vi "MU Read Sens.vi"(8 "error in (no error)":errorcluster, 11 "handle":u64) -> (0 "error out (no error)":errorcluster, 2 "data":T1, 3 "function return":u32)   [LabVIEW 2017, in "MU_3SL_interface.lvlib"]
uses:
  MU_3SL_interface.lvlib
  lib/MU_3SL_interface.dll
panel:
  in  "data":T1
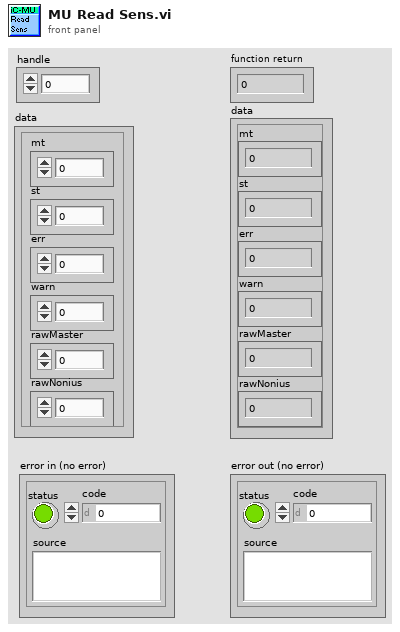
[diagram p1: front panel]
types:
  T1 = cluster{"mt":u32, "st":u32, "err":u32, "warn":u32, "rawMaster":u32, "rawNonius":u32}
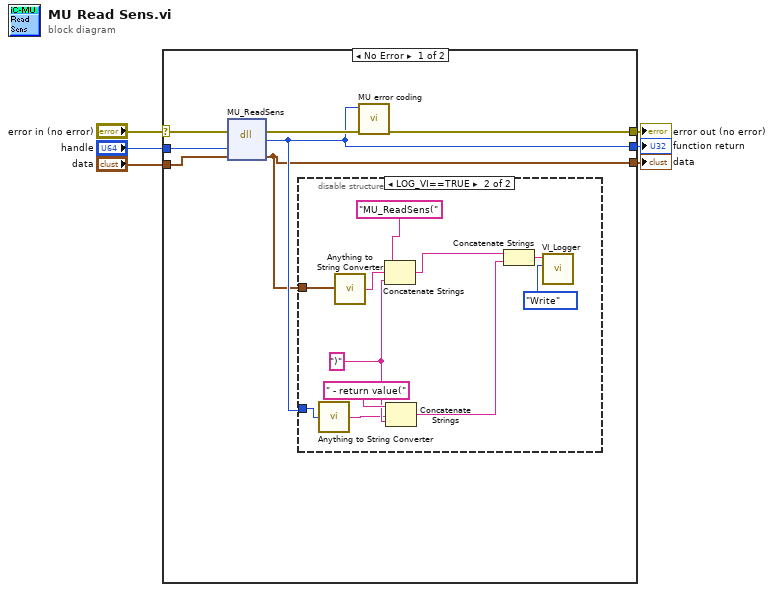
[diagram p0: block diagram]
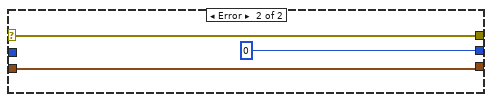
[diagram p3: hidden frame]
diagram:
  n1 = case shown="No Error" "error in (no error)" {
    selector: "error in (no error)" -> [w9 w27]
    tunnel: [w8 u32 0 ("return type")] -> w6
    tunnel: "handle" -> [w13 _]
    tunnel: [w11 w27] -> w4
    tunnel: "data" -> [w10 w25]
    tunnel: [w7 w25] -> w1
    frame No Error {
      n2 = dll-call lib="C:/Users/bes/AppData/Roaming/work/mu_9so/icsubmodules/soft_mu_3sl_master/lv_interface/lib/MU_3SL_interface**.*" fn="MU_ReadSens"(error in=w9, "handle"=w13, "data"=w10) -> (error out=w12:errorcluster, "return type"=w8:u32, "data"=w7:T1)  [unwired: 3 in, 1 out]
      n3 = disable-structure shown="LOG_VI==TRUE" {
        disable-tunnel: w8 -> [_ w16]
        disable-tunnel: w7 -> [_ w18]
        frame condition #0 {
        }
        frame condition #1 (active) {
          w19 = ")" ("string")
          n4 = call "Anything to String Converter.vi"("anything"=w16) -> ("String"=w15:string)
          n5 = call "Anything to String Converter.vi"("anything"=w18) -> ("String"=w17:string)
          n6 = Concatenate Strings("MU_ReadSens(" ("Info in"), w17, w19) -> (w14:string)
          n7 = Concatenate Strings(" - return value(" ("string"), w15, w19) -> (w22:string)
          n8 = Concatenate Strings(w14, w22) -> (w21:string)
          n9 = call "VI_Logger.vi"("Action (Read)"=enum16{"Write", "Read"}."Write", "Info in"=w21) -> ()  [unwired: 8 in, 2 out]
        }
      }
      n10 = call "MU error coding.vi"("error in (no error)"=w12, "function return in"=w8) -> ("error out"=w11:errorcluster)  [unwired: 9 in]
    }
    frame Error {
    }
  }
  "function return" <- w6
  "error out (no error)" <- w4
  "data" <- w1
